vi "Check for lock-in.vi"() -> (1 "SR830 lock-in detected":bool, 3 "VISA resource name":refnum<visa-resource-name>)   [LabVIEW 2012, in "SR830.lvlib"]
doc: "Checks to see if a Stanford Research Systems SR830 DSP lock-in amplifier is connected to the computer and returns true or false, along with the VISA resource name if true."
uses:
  SR830.lvlib
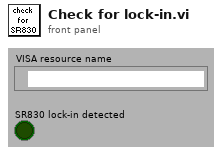
[diagram p1: front panel]
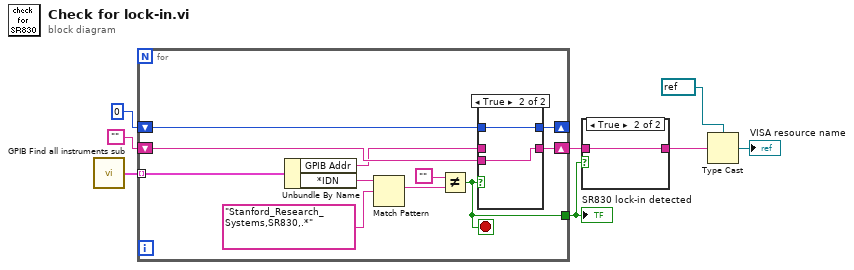
[diagram p0: block diagram]
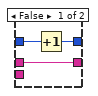
[diagram p2: hidden frame]
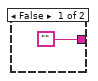
[diagram p3: hidden frame]
diagram:
  n1 = call "GPIB Find all instruments sub.vi"() -> ("Array"=w3:cluster{"GPIB Addr":string, "*IDN":string}[])
  n2 = for {
    tunnel: w3 -> [w19] mode=indexing
    shift-right: [w15] -> _
    shift-left: 0 -> [w16]
    shift-right: [w17] -> w4
    shift-left: "" -> [w13]
    tunnel: [w9] -> w2
    stop <- w9 stop-if-true
    n3 = Unbundle By Name(w19) -> ("GPIB Addr"=w11:string, "*IDN"=w12:string)
    n4 = Match Pattern(string=w12, regular expression="Stanford_Research_Systems,SR830,.*") -> (match substring=w14:string)  [unwired: 4 out]
    n5 = Not Equal?(x="", y=w14) -> (x != y?=w9:bool)
    n6 = case shown="True" w9 {
      tunnel: [w22 w23] -> w17
      tunnel: w11 -> [w22 _]
      tunnel: w16 -> [w21 w24]
      tunnel: [w20 w24] -> w15
      tunnel: w13 -> [_ w23]
      frame False {
        n7 = Increment(x=w21) -> (x+1=w20:i32)
      }
      frame True {
      }
    }
  }
  "SR830 lock-in detected" <- w2
  n8 = case shown="True" w2 {
    tunnel: w4 -> [_ w26]
    tunnel: ["" w26] -> w6
    frame False {
    }
    frame True {
    }
  }
  n9 = Type Cast(type=refnum<visa-resource-name> refnum ("VISA resource name"), x=w6) -> (*(type *) &x=→"VISA resource name":refnum<visa-resource-name>)
